vi "IO.vi"() -> ()   [LabVIEW 2020]
uses:
  Global_Variable/Global.vi
  Libraries/S7/S7.lvlib
panel:
  in  "输入轴旋转手动速度":sgl caption="手动速度" format="%#.3f"
  in  "输入轴旋转-正转":bool
  in  "输入轴旋转-反转":bool
  in  "输入轴旋转绝对位置":sgl caption="绝对位置" format="%#.3f"
  in  "输入轴旋转相对位置":sgl caption="相对位置" format="%#.3f"
  in  "输入轴旋转-绝对定位":bool
  in  "输入轴旋转-相对定位":bool
  out "输出轴旋转当前位置":sgl caption="当前位置" format="%#.3f"
  in  "输出轴旋转-反转":bool
  in  "输出轴旋转-正转":bool
  in  "输出轴旋转手动速度":sgl caption="手动速度" format="%#.3f"
  in  "工装移载手动速度":sgl caption="手动速度" format="%#.3f"
  in  "工装移载-正转":bool
  in  "工装移载-反转":bool
  in  "工装移载绝对位置":sgl caption="绝对位置" format="%#.3f"
  in  "工装移载相对位置":sgl caption="相对位置" format="%#.3f"
  in  "工装移载-绝对定位":bool
  in  "工装移载-相对定位":bool
  out "输入轴旋转状态":bool
  out "工装移载状态":bool
  out "输出轴旋转状态":bool
  in  "选项卡控件":enum32{"DI", "DO", "伺服"}(tab)
  out "I 1":T1
  out "I 3":T2
  out "I 2":T3
  out "I 0":T4
  out "I 4":T5
  out "I 5":T6
  in  "Q5":T7
  in  "Q4":T8
  in  "Q3":T9
  in  "Q2":T10
  in  "Q1":T11
  in  "Q0":T12
  out "电机角度":sgl caption="电机角度(°)" format="%#.3f"
  out "扭矩":sgl caption="扭矩(N)" format="%#.3f"
  out "拉压力":sgl caption="拉压力(N)" format="%#.3f"
  in  "输入轴移载相对位置":sgl caption="相对位置" format="%#.3f"
  in  "输入轴移载绝对位置":sgl caption="绝对位置" format="%#.3f"
  in  "拧紧轴手动速度":sgl caption="手动速度" format="%#.3f"
  out "输入轴移载状态":bool
  in  "输入轴移载-相对定位":bool
  in  "输入轴移载-绝对定位":bool
  in  "拧紧轴-反转":bool
  in  "拧紧轴-正转":bool
  out "输入轴旋转当前位置":sgl caption="当前位置" format="%#.3f"
  out "输入轴移载当前位置":sgl caption="当前位置" format="%#.3f"
  out "工装移载当前位置":sgl caption="当前位置" format="%#.3f"
  out "位移":sgl caption="电缸位移(MM)" format="%#.3f"
  in  "Q6":T13
  # "手动操作"
  # "输入轴旋转伺服"
  # "输出轴旋转伺服"
  # "工装移载伺服"
  # "输入轴移载伺服"
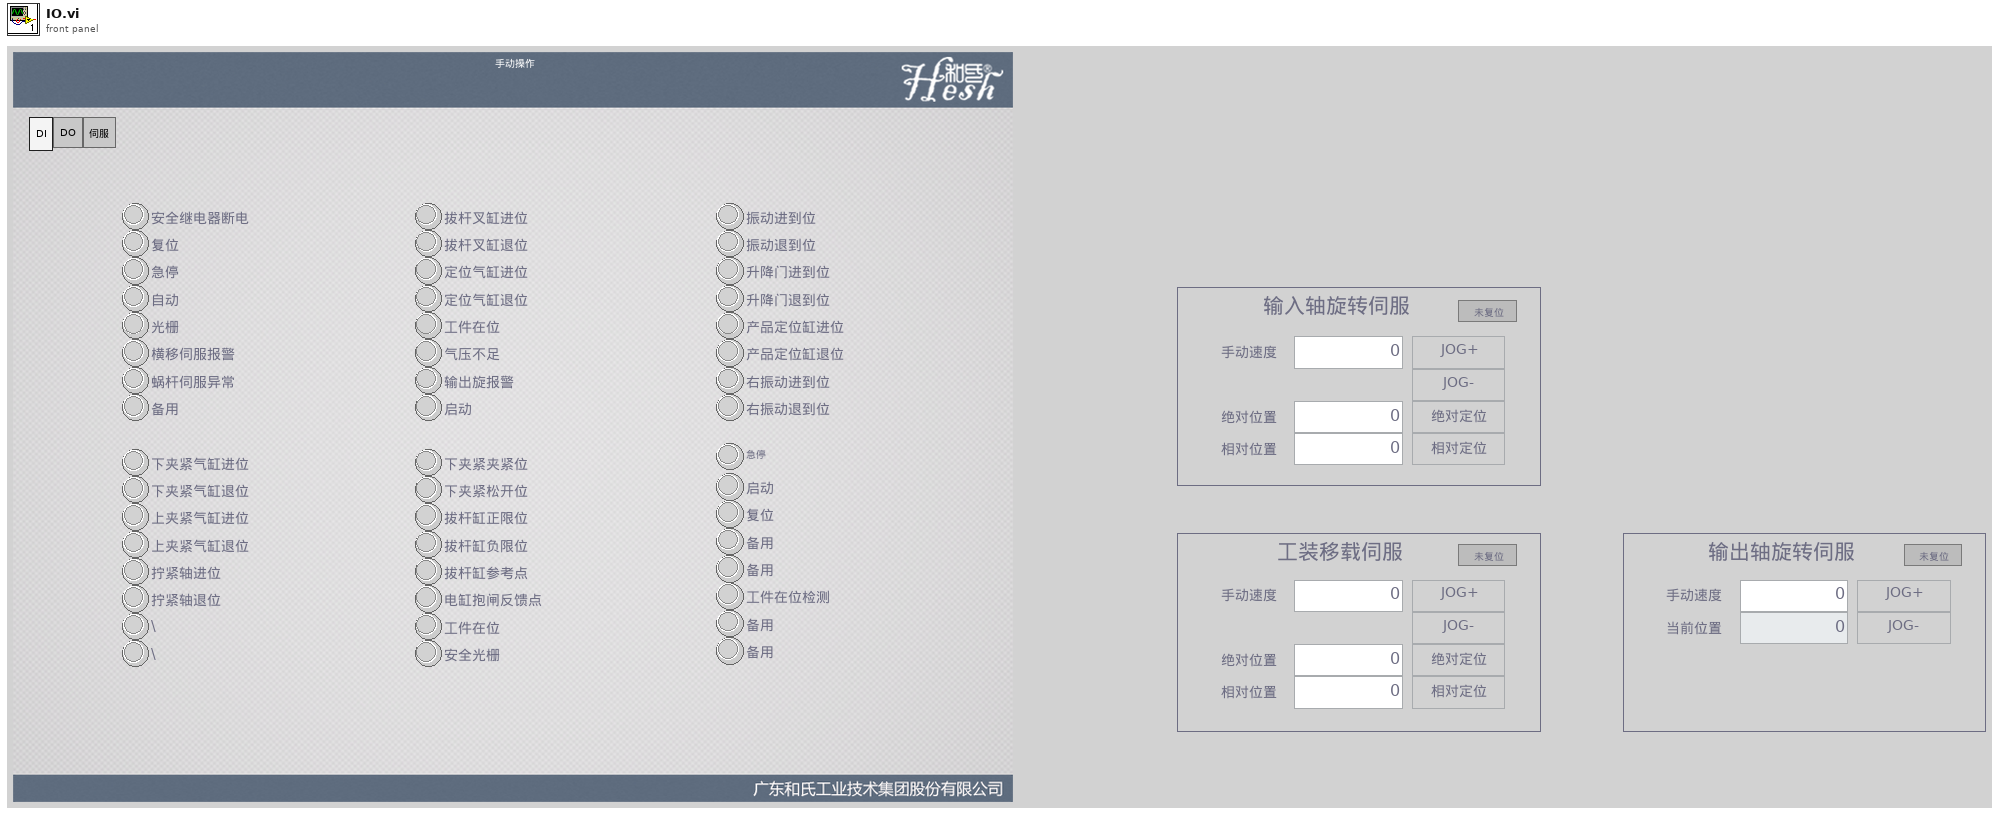
[diagram p1: front panel]
types:
  T1 = cluster{"下夹紧气缸进位":bool, "下夹紧气缸退位":bool, "上夹紧气缸进位":bool, "上夹紧气缸退位":bool, "拧紧轴进位":bool, "拧紧轴退位":bool, "\\":bool, "\\ ":bool}
  T2 = cluster{"下夹紧夹紧位":bool, "下夹紧松开位":bool, "拔杆缸正限位":bool, "拔杆缸负限位":bool, "拔杆缸参考点":bool, "电缸抱闸反馈点":bool, "工件在位":bool, "安全光栅":bool}
  T3 = cluster{"拔杆叉缸进位":bool, "拔杆叉缸退位":bool, "定位气缸进位":bool, "定位气缸退位":bool, "工件在位":bool, "气压不足":bool, "输出旋报警":bool, "启动":bool}
  T4 = cluster{"安全继电器断电":bool, "复位":bool, "急停":bool, "自动":bool, "光栅":bool, "横移伺服报警":bool, "蜗杆伺服异常":bool, "备用":bool}
  T5 = cluster{"振动进到位":bool, "振动退到位":bool, "升降门进到位":bool, "升降门退到位":bool, "产品定位缸进位":bool, "产品定位缸退位":bool, "右振动进到位":bool, "右振动退到位":bool}
  T6 = cluster{"急停":bool, "启动":bool, "复位":bool, "备用":bool, "备用":bool, "工件在位检测":bool, "备用":bool, "备用":bool}
  T7 = cluster{"产品定位缸进":bool, "产品定位缸退":bool, "右振动进":bool, "右振动退":bool, "高度适配轴复位":bool, "高度适配轴回原点":bool, "高度适配轴JOG+":bool, "高度适配轴JOG-":bool}
  T8 = cluster{"抱花键":bool, "摆臂进":bool, "摆臂退":bool, "升降门进":bool, "升降门退":bool, "振动":bool, "电机方向":bool, "电机控制":bool}
  T9 = cluster{"定位缸进":bool, "定位缸退":bool, "三色灯红":bool, "蜂鸣器":bool, "备用":bool, "switch":bool, "备用":bool, "备用":bool}
  T10 = cluster{"下气缸夹紧":bool, "下气缸松开":bool, "上气缸夹紧":bool, "上气缸松开":bool, "拧紧轴进":bool, "拧紧轴退":bool, "拔叉缸进":bool, "拔叉缸退":bool}
  T11 = cluster{"合格":bool, "不合格":bool, "/":bool, "/":bool, "/":bool, "/":bool, "/":bool, "/":bool}
  T12 = cluster{"轴1上":bool, "轴1下":bool, "轴2脉冲":bool, "轴2方向":bool, "蜂鸣器":bool, "黄灯":bool, "绿灯":bool, "红灯":bool}
  T13 = cluster{"输入轴移载上升":bool, "输入轴移载下降":bool, "输出轴移载上升":bool, "输出轴移载下降":bool, "输入轴左旋":bool, "输入轴右旋":bool, "输出轴左旋":bool, "输出轴右旋":bool}
  T14 = cluster{bool, bool, bool, bool, bool, bool, bool, bool}
  T15 = typedef "S7.lvlib/Read_Data (Reply Payload)--cluster.ctl" = cluster{"读取成功":bool, "数据":u32[], "Read_Data_error":errorcluster}
  T16 = cluster{"Boolean array[0]":bool, "Boolean array[1]":bool, "Boolean array[2]":bool, "Boolean array[3]":bool, "Boolean array[4]":bool, "Boolean array[5]":bool, "Boolean array[6]":bool, "Boolean array[7]":bool}
  T17 = cluster{"输入旋转位移":sgl, "输入移载位移":sgl, "工装移载位移":sgl, "输入编码位移":sgl, "扭矩":sgl, "输出扭矩(小)":sgl, "输出扭矩(大)":sgl, "吸收电流":sgl, "Factorysensor":sgl, "输出轴旋转角度":sgl, "输出轴移栽位移":sgl, "Factorysensor2":sgl}
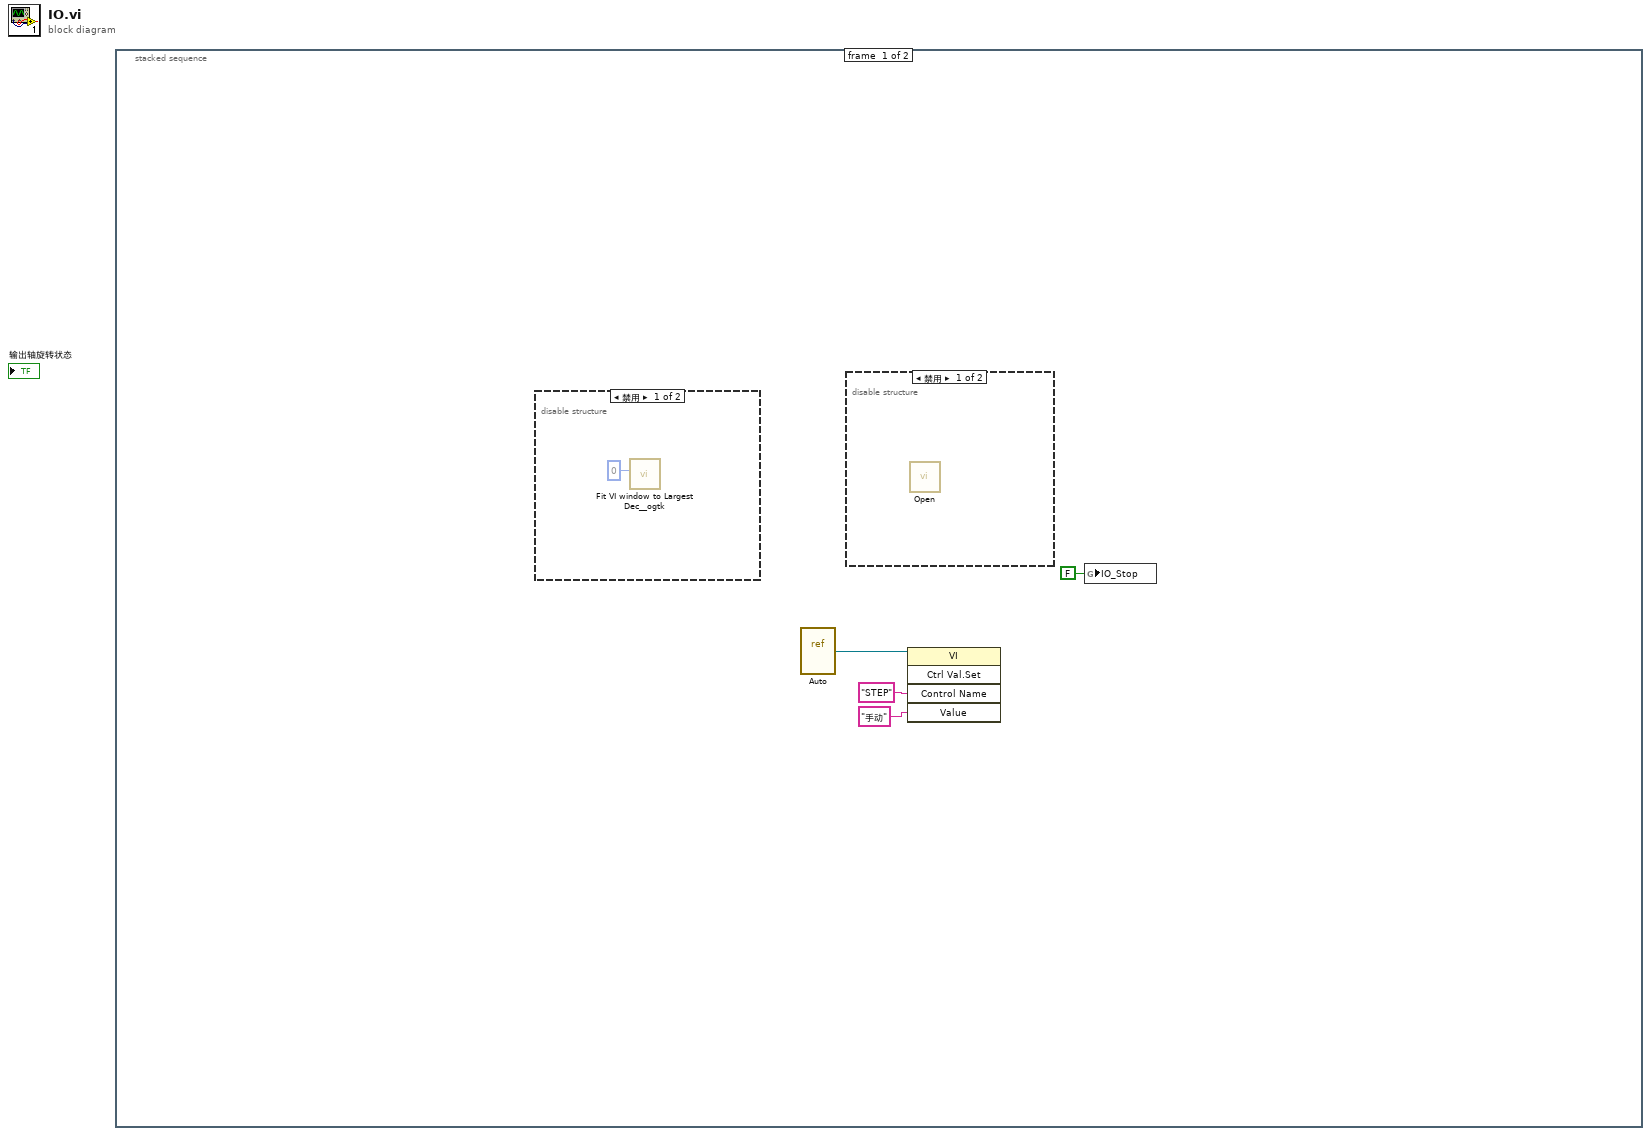
[diagram p0: block diagram]
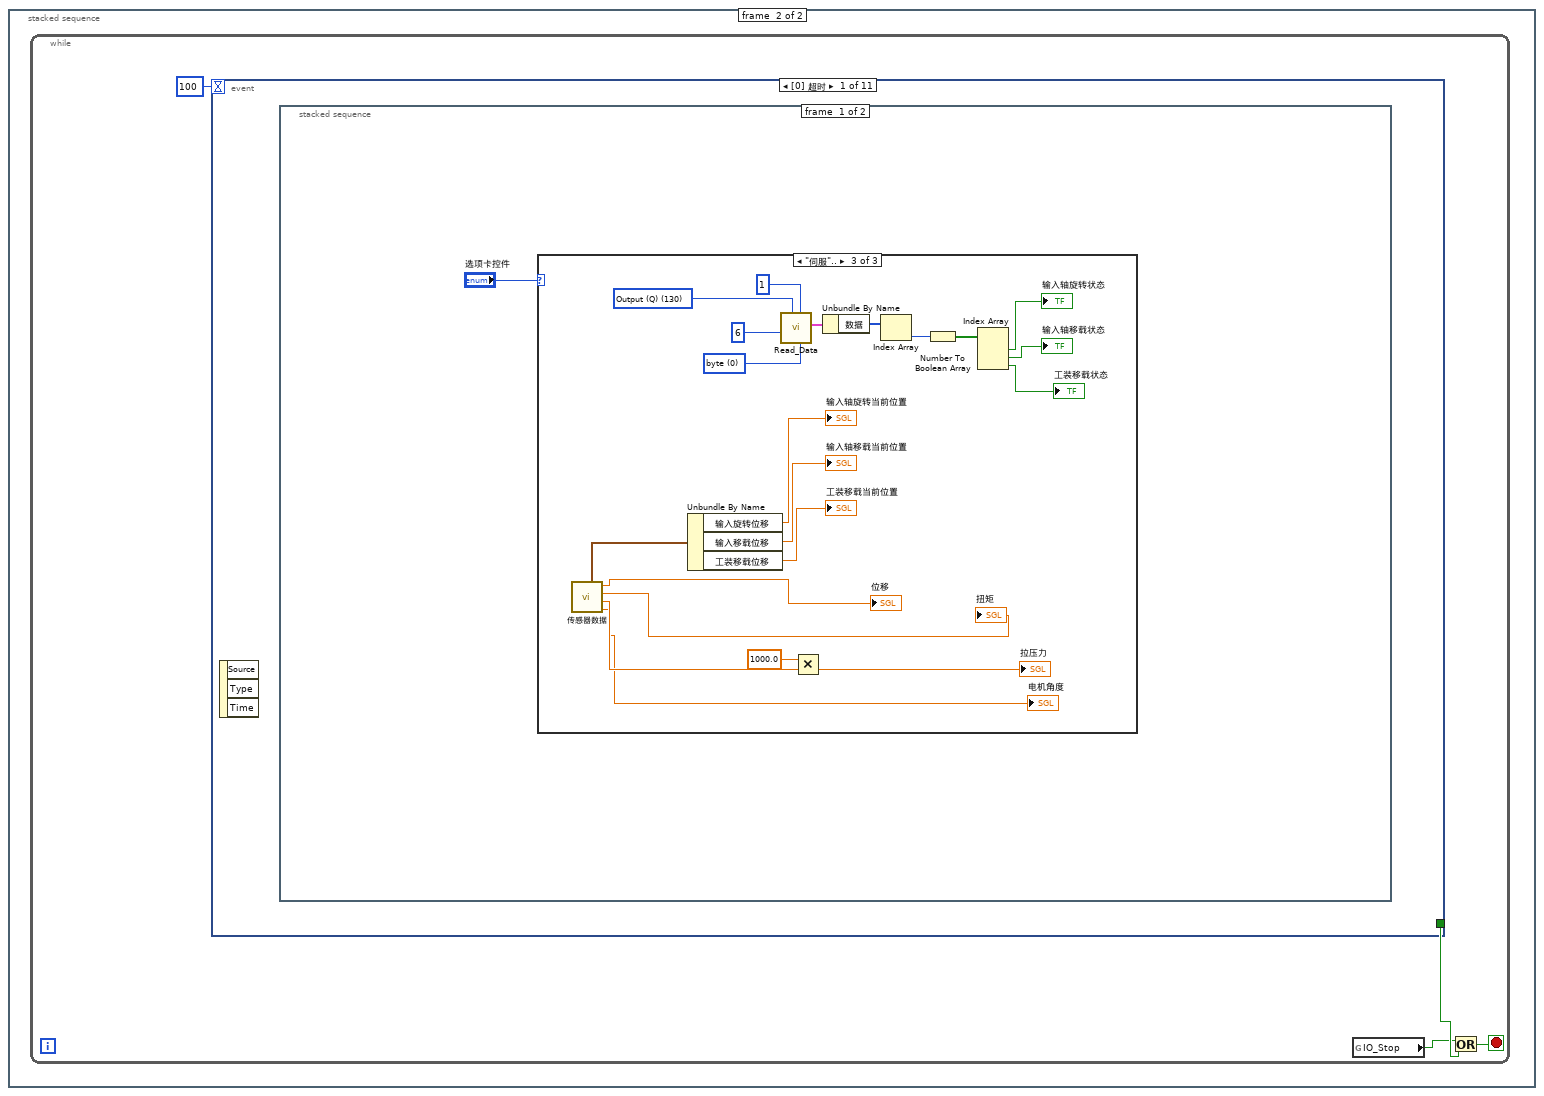
[diagram p4: hidden frame]
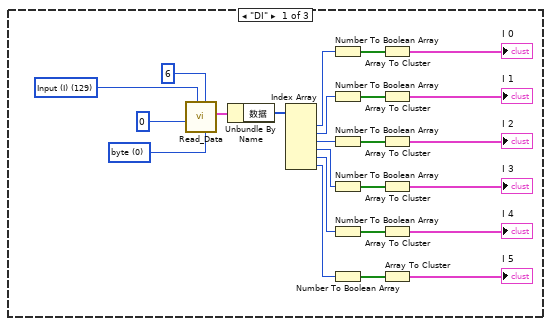
[diagram p5: hidden frame]
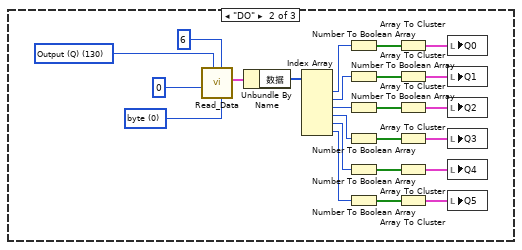
[diagram p6: hidden frame]
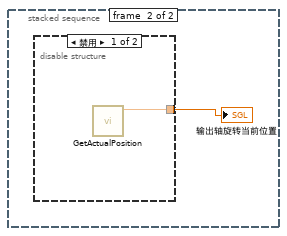
[diagram p7: hidden frame]
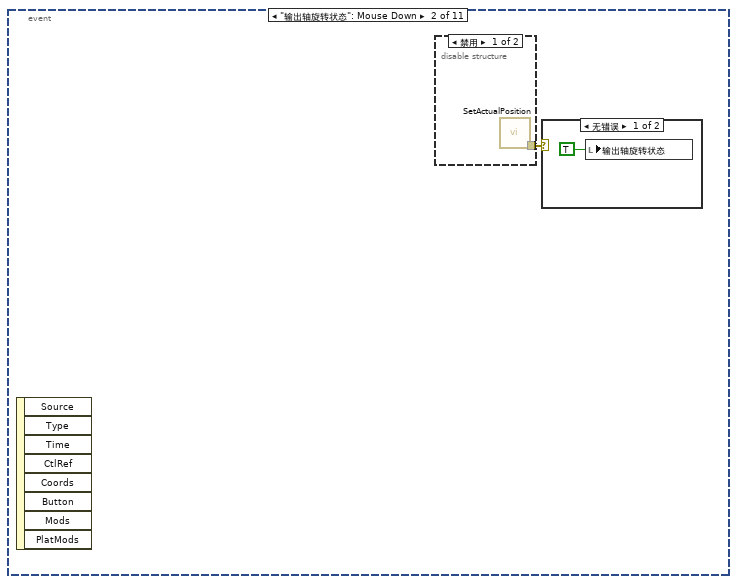
[diagram p9: hidden frame]
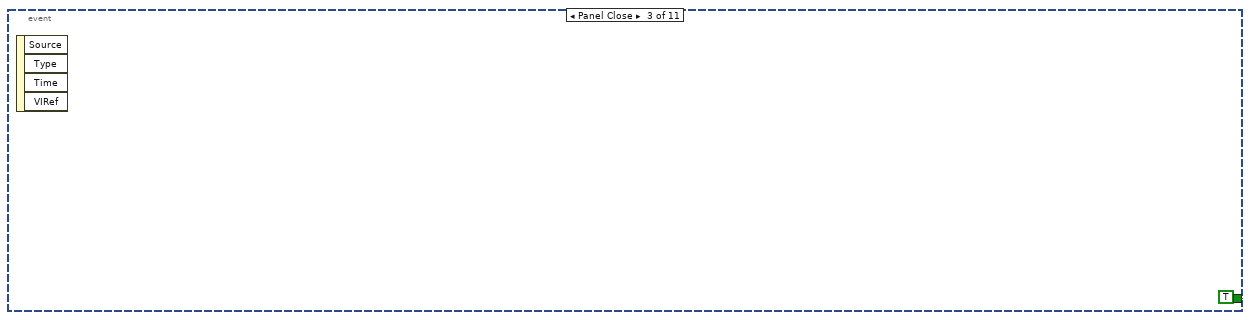
[diagram p12: hidden frame]
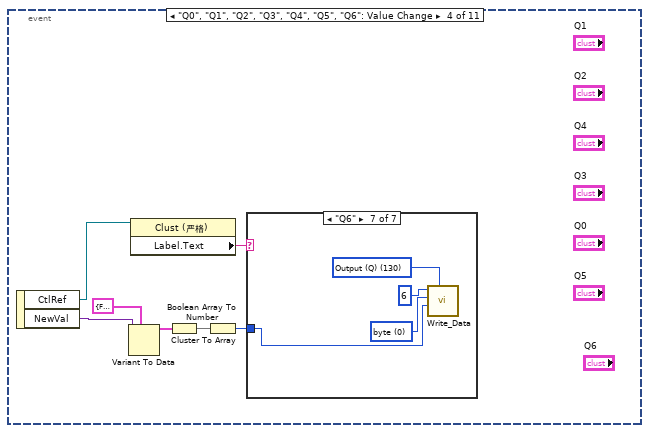
[diagram p13: hidden frame]
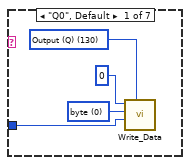
[diagram p14: hidden frame]
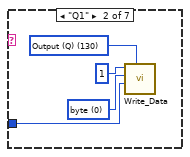
[diagram p15: hidden frame]
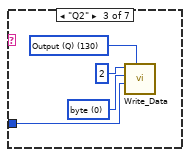
[diagram p16: hidden frame]
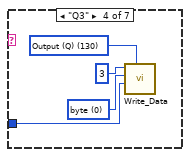
[diagram p17: hidden frame]
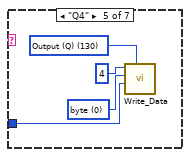
[diagram p18: hidden frame]
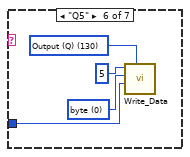
[diagram p19: hidden frame]
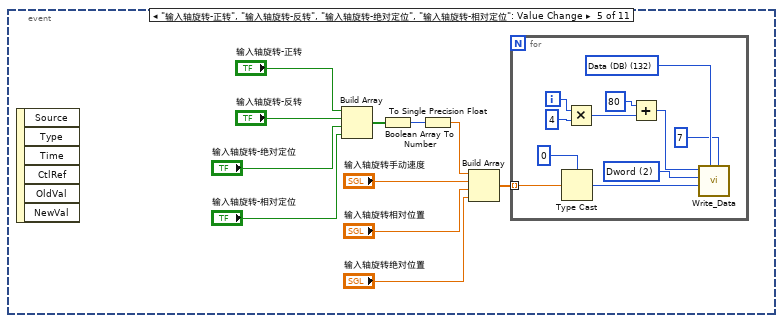
[diagram p20: hidden frame]
diagram:
  n1 = stacked-sequence {
    frame #0 {
      n2 = disable-structure shown="禁用" {
        frame Disabled {
          n3 = call <userlib>:"Fit VI window to Largest Dec__ogtk.vi"("border spacing (2 px)"=0) -> ()  [unwired: 5 in, 2 out]
        }
        frame Enabled {
        }
      }
      n4 = vi-ref "Auto.vi"() -> (w3:refnum<vi>)
      n5 = disable-structure shown="禁用" {
        frame Disabled {
          n6 = call "Open.vi"() -> ()  [unwired: 11 in, 1 out]
        }
        frame Enabled {
        }
      }
      n7 = invoke class="VI" method="Ctrl Val.Set"(reference=w3, "Control Name"="STEP" ("控件名"), "Value"="手动" ("控件名")) -> ()  [unwired: 2 in, 5 out]
      n8 = global write "Global.vi" "IO_Stop"(FALSE ("IO_Stop")) -> ()
    }
    frame #1 {
      n9 = while {
        stop <- w6 stop-if-true
        n10 = event shown="[0] 超时" {
          selector: _ -> [_ _ _ _ _ _ _ _ _ _ _]
          dyn-events: _ -> [_ _ _ _ _ _ _ _ _ _ _]
          timeout: 100 -> [_ _ _ _ _ _ _ _ _ _ _]
          tunnel: [_ _ TRUE _ _ _ _ _ _ _ _] -> w8
          event Timeout {
            n11 = event-data() -> ()  [unwired: 1 in, 3 out]
            n12 = stacked-sequence {
              frame #0 {
                n13 = case shown="\"伺服\".." "选项卡控件" {
                  frame "DI" {
                    w14 = u16 0 items=["byte", "word", "Dword"] ("数据类型")
                    w12 = u8 129 items=["I/O (P)"=128, "Input (I)"=129, "Output (Q)"=130, "Bit Memory (M)"=131, "Data (DB)"=132, "Instance Data (DI)"=133, "Local Data (L)"=134, "Predecessor Local Data (VL)"=135] ("寄存器类型")
                    n14 = call "Read_Data.vi"("数据类型"=w14, "读取长度"=u16 6, "寄存器类型"=w12, "起始地址"=u32 0) -> ("Reply Payload"=w16:T15)  [unwired: 5 in, 2 out]
                    n15 = Unbundle By Name(w16) -> ("数据"=w15:u32[])
                    n16 = Index Array(array=w15) -> (element #1=w28:u32, element #2=w30:u32, element #3=w29:u32, element #4=w25:u32, element #5=w24:u32, element #6=w23:u32)  [unwired: 6 in]
                    n17 = Number To Boolean Array(number=w28) -> (Boolean array=w27:bool[])
                    n18 = Number To Boolean Array(number=w30) -> (Boolean array=w26:bool[])
                    n19 = Number To Boolean Array(number=w29) -> (Boolean array=w22:bool[])
                    n20 = Number To Boolean Array(number=w25) -> (Boolean array=w20:bool[])
                    n21 = Number To Boolean Array(number=w24) -> (Boolean array=w18:bool[])
                    n22 = Number To Boolean Array(number=w23) -> (Boolean array=w17:bool[])
                    n23 = Array To Cluster(array=w27) -> (cluster=→"I 0":T16)
                    n24 = Array To Cluster(array=w26) -> (cluster=→"I 1":T16)
                    n25 = Array To Cluster(array=w22) -> (cluster=→"I 2":T16)
                    n26 = Array To Cluster(array=w20) -> (cluster=→"I 3":T16)
                    n27 = Array To Cluster(array=w18) -> (cluster=→"I 4":T16)
                    n28 = Array To Cluster(array=w17) -> (cluster=→"I 5":T16)
                  }
                  frame "DO" {
                    w38 = u16 0 items=["byte", "word", "Dword"] ("数据类型")
                    w36 = u8 130 items=["I/O (P)"=128, "Input (I)"=129, "Output (Q)"=130, "Bit Memory (M)"=131, "Data (DB)"=132, "Instance Data (DI)"=133, "Local Data (L)"=134, "Predecessor Local Data (VL)"=135] ("寄存器类型")
                    n29 = call "Read_Data.vi"("数据类型"=w38, "读取长度"=u16 6, "寄存器类型"=w36, "起始地址"=u32 0) -> ("Reply Payload"=w57:T15)  [unwired: 5 in, 2 out]
                    n30 = Unbundle By Name(w57) -> ("数据"=w58:u32[])
                    n31 = Index Array(array=w58) -> (element #1=w48:u32, element #2=w50:u32, element #3=w49:u32, element #4=w47:u32, element #5=w46:u32, element #6=w45:u32)  [unwired: 6 in]
                    n32 = Number To Boolean Array(number=w48) -> (Boolean array=w51:bool[])
                    n33 = Number To Boolean Array(number=w50) -> (Boolean array=w52:bool[])
                    n34 = Number To Boolean Array(number=w49) -> (Boolean array=w53:bool[])
                    n35 = Number To Boolean Array(number=w47) -> (Boolean array=w54:bool[])
                    n36 = Number To Boolean Array(number=w46) -> (Boolean array=w55:bool[])
                    n37 = Number To Boolean Array(number=w45) -> (Boolean array=w56:bool[])
                    n38 = Array To Cluster(array=w51) -> (cluster=w43:T16)
                    n39 = Array To Cluster(array=w52) -> (cluster=w44:T16)
                    n40 = Array To Cluster(array=w53) -> (cluster=w41:T16)
                    n41 = Array To Cluster(array=w54) -> (cluster=w42:T16)
                    n42 = Array To Cluster(array=w55) -> (cluster=w40:T16)
                    n43 = Array To Cluster(array=w56) -> (cluster=w39:T16)
                    n44 = local write "Q0"(w43) -> ()
                    n45 = local write "Q1"(w44) -> ()
                    n46 = local write "Q2"(w41) -> ()
                    n47 = local write "Q3"(w42) -> ()
                    n48 = local write "Q4"(w40) -> ()
                    n49 = local write "Q5"(w39) -> ()
                  }
                  frame "伺服".. {
                    w72 = u16 0 items=["byte", "word", "Dword"] ("数据类型")
                    w70 = u8 130 items=["I/O (P)"=128, "Input (I)"=129, "Output (Q)"=130, "Bit Memory (M)"=131, "Data (DB)"=132, "Instance Data (DI)"=133, "Local Data (L)"=134, "Predecessor Local Data (VL)"=135] ("寄存器类型")
                    n50 = call "传感器数据.vi"() -> ("电机角度"=→"电机角度":sgl, "拉压力"=w64:sgl, "扭矩"=→"扭矩":sgl, "电缸位移"=→"位移":sgl, "传感器读数"=w60:T17)  [unwired: 6 in, 1 out]
                    n51 = Unbundle By Name(w60) -> ("输入旋转位移"=→"输入轴旋转当前位置":sgl, "输入移载位移"=→"输入轴移载当前位置":sgl, "工装移载位移"=→"工装移载当前位置":sgl)
                    n52 = call "Read_Data.vi"("数据类型"=w72, "读取长度"=u16 1, "寄存器类型"=w70, "起始地址"=u32 6) -> ("Reply Payload"=w73:T15)  [unwired: 5 in, 2 out]
                    n53 = Multiply(x=sgl 1000.0, y=w64) -> (x*y=→"拉压力":sgl)
                    n54 = Unbundle By Name(w73) -> ("数据"=w74:u32[])
                    n55 = Index Array(array=w74) -> (element=w79:u32)  [unwired: 1 in]
                    n56 = Number To Boolean Array(number=w79) -> (Boolean array=w76:bool[])
                    n57 = Index Array(array=w76) -> (element #1=→"输入轴旋转状态":bool, element #2=→"输入轴移载状态":bool, element #3=→"工装移载状态":bool)  [unwired: 3 in]
                  }
                }
              }
              frame #1 {
                n58 = disable-structure shown="禁用" {
                  disable-tunnel: [w81 _] -> w80
                  frame Disabled {
                    n59 = call "GetActualPosition.vi"() -> ("Axis_ActualPosition(°)"=w81:dbl)  [unwired: 11 in]
                  }
                  frame Enabled {
                  }
                }
                "输出轴旋转当前位置" <- w80
              }
            }
          }
          event "输出轴旋转状态": Mouse Down {
            n60 = event-data() -> ()  [unwired: 1 in, 8 out]
            n61 = disable-structure shown="禁用" {
              disable-tunnel: [w83 _] -> w82
              frame Disabled {
                n62 = call "SetActualPosition.vi"() -> ("error out"=w83:errorcluster)  [unwired: 11 in]
              }
              frame Enabled {
              }
            }
            n63 = case shown="无错误" w82 {
              frame No Error {
                n64 = local write "输出轴旋转状态"(TRUE ("输出轴旋转状态")) -> ()
              }
              frame Error {
              }
            }
          }
          event Panel Close {
            n65 = event-data() -> ()  [unwired: 1 in, 4 out]
          }
          event "Q0", "Q1", "Q2", "Q3", "Q4", "Q5", "Q6": Value Change {
            n66 = event-data() -> ("CtlRef"=w87:refnum<vi>, "NewVal"=w91:variant)  [unwired: 1 in]
            n67 = Variant To Data(type=T14 {FALSE, FALSE, FALSE, FALSE, FALSE, FALSE, FALSE, FALSE}, Variant=w91) -> (data=w90:T14)  [unwired: 1 in, 1 out]
            n68 = property class="Clust (严格)"(reference=w87) -> ("Label.Text"=w86:string)  [unwired: 1 in, 2 out]
            n69 = Cluster To Array(cluster=w90) -> (array=w89:bool[])
            n70 = Boolean Array To Number(Boolean array=w89) -> (number=w88:u32)
            n71 = case shown="\"Q6\"" w86 {
              tunnel: w88 -> [w96 w100 w104 w108 w112 w116 w117]
              frame "Q0", Default {
                w94 = u16 0 items=["byte", "word", "Dword"] ("数据类型")
                w95 = u8 130 items=["I/O (P)"=128, "Input (I)"=129, "Output (Q)"=130, "Bit Memory (M)"=131, "Data (DB)"=132, "Instance Data (DI)"=133, "Local Data (L)"=134, "Predecessor Local Data (VL)"=135] ("寄存器类型")
                n72 = call "Write_Data.vi"("寄存器类型"=w95, "写入数据"=w96, "数据类型"=w94, "写入地址"=u32 0) -> ()  [unwired: 5 in, 3 out]
              }
              frame "Q1" {
                w98 = u16 0 items=["byte", "word", "Dword"] ("数据类型")
                w99 = u8 130 items=["I/O (P)"=128, "Input (I)"=129, "Output (Q)"=130, "Bit Memory (M)"=131, "Data (DB)"=132, "Instance Data (DI)"=133, "Local Data (L)"=134, "Predecessor Local Data (VL)"=135] ("寄存器类型")
                n73 = call "Write_Data.vi"("寄存器类型"=w99, "写入数据"=w100, "数据类型"=w98, "写入地址"=u32 1) -> ()  [unwired: 5 in, 3 out]
              }
              frame "Q2" {
                w102 = u16 0 items=["byte", "word", "Dword"] ("数据类型")
                w103 = u8 130 items=["I/O (P)"=128, "Input (I)"=129, "Output (Q)"=130, "Bit Memory (M)"=131, "Data (DB)"=132, "Instance Data (DI)"=133, "Local Data (L)"=134, "Predecessor Local Data (VL)"=135] ("寄存器类型")
                n74 = call "Write_Data.vi"("寄存器类型"=w103, "写入数据"=w104, "数据类型"=w102, "写入地址"=u32 2) -> ()  [unwired: 5 in, 3 out]
              }
              frame "Q3" {
                w106 = u16 0 items=["byte", "word", "Dword"] ("数据类型")
                w107 = u8 130 items=["I/O (P)"=128, "Input (I)"=129, "Output (Q)"=130, "Bit Memory (M)"=131, "Data (DB)"=132, "Instance Data (DI)"=133, "Local Data (L)"=134, "Predecessor Local Data (VL)"=135] ("寄存器类型")
                n75 = call "Write_Data.vi"("寄存器类型"=w107, "写入数据"=w108, "数据类型"=w106, "写入地址"=u32 3) -> ()  [unwired: 5 in, 3 out]
              }
              frame "Q4" {
                w110 = u16 0 items=["byte", "word", "Dword"] ("数据类型")
                w111 = u8 130 items=["I/O (P)"=128, "Input (I)"=129, "Output (Q)"=130, "Bit Memory (M)"=131, "Data (DB)"=132, "Instance Data (DI)"=133, "Local Data (L)"=134, "Predecessor Local Data (VL)"=135] ("寄存器类型")
                n76 = call "Write_Data.vi"("寄存器类型"=w111, "写入数据"=w112, "数据类型"=w110, "写入地址"=u32 4) -> ()  [unwired: 5 in, 3 out]
              }
              frame "Q5" {
                w114 = u16 0 items=["byte", "word", "Dword"] ("数据类型")
                w115 = u8 130 items=["I/O (P)"=128, "Input (I)"=129, "Output (Q)"=130, "Bit Memory (M)"=131, "Data (DB)"=132, "Instance Data (DI)"=133, "Local Data (L)"=134, "Predecessor Local Data (VL)"=135] ("寄存器类型")
                n77 = call "Write_Data.vi"("寄存器类型"=w115, "写入数据"=w116, "数据类型"=w114, "写入地址"=u32 5) -> ()  [unwired: 5 in, 3 out]
              }
              frame "Q6" {
                w119 = u16 0 items=["byte", "word", "Dword"] ("数据类型")
                w120 = u8 130 items=["I/O (P)"=128, "Input (I)"=129, "Output (Q)"=130, "Bit Memory (M)"=131, "Data (DB)"=132, "Instance Data (DI)"=133, "Local Data (L)"=134, "Predecessor Local Data (VL)"=135] ("寄存器类型")
                n78 = call "Write_Data.vi"("寄存器类型"=w120, "写入数据"=w117, "数据类型"=w119, "写入地址"=u32 6) -> ()  [unwired: 5 in, 3 out]
              }
            }
          }
          event "输入轴旋转-正转", "输入轴旋转-反转", "输入轴旋转-绝对定位", "输入轴旋转-相对定位": Value Change {
            n79 = event-data() -> ()  [unwired: 1 in, 6 out]
            n80 = Build Array("输入轴旋转-正转", "输入轴旋转-反转", "输入轴旋转-绝对定位", "输入轴旋转-相对定位") -> (w130:bool[])
            n81 = Boolean Array To Number(Boolean array=w130) -> (number=w129:u32)
            n82 = To Single Precision Float(number=w129) -> (single precision float=w131:sgl)
            n83 = Build Array(w131, "输入轴旋转手动速度", "输入轴旋转相对位置", "输入轴旋转绝对位置") -> (w128:sgl[])
            n84 = for {
              tunnel: w128 -> [w137] mode=indexing
              i -> [w134]
              w139 = u16 2 items=["byte", "word", "Dword"] ("数据类型")
              w142 = u8 132 items=["I/O (P)"=128, "Input (I)"=129, "Output (Q)"=130, "Bit Memory (M)"=131, "Data (DB)"=132, "Instance Data (DI)"=133, "Local Data (L)"=134, "Predecessor Local Data (VL)"=135] ("寄存器类型")
              n85 = Type Cast(type=u32 0, x=w137) -> (*(type *) &x=w136:u32)
              n86 = Multiply(x=w134, y=u32 4) -> (x*y=w133:u32)
              n87 = Add(x=u32 80 ("写入地址"), y=w133) -> (x+y=w132:u32)
              n88 = call "Write_Data.vi"("DB #"=u16 7, "寄存器类型"=w142, "写入数据"=w136, "数据类型"=w139, "写入地址"=w132) -> ()  [unwired: 4 in, 3 out]
            }
          }
          event "拧紧轴-正转", "拧紧轴-反转", "输入轴移载-绝对定位", "输入轴移载-相对定位": Value Change {
            n89 = event-data() -> ()  [unwired: 1 in, 6 out]
            n90 = Build Array("拧紧轴-正转", "拧紧轴-反转", "输入轴移载-绝对定位", "输入轴移载-相对定位") -> (w152:bool[])
            n91 = Boolean Array To Number ("布尔数组至数值转换")(Boolean array=w152) -> (number=w151:u32)
            n92 = To Single Precision Float ("转换为单精度浮点数")(number=w151) -> (single precision float=w153:sgl)
            n93 = Build Array(w153, "拧紧轴手动速度", "输入轴移载相对位置", "输入轴移载绝对位置") -> (w150:sgl[])
            n94 = for {
              tunnel: w150 -> [w162] mode=indexing
              i -> [w160]
              w155 = u16 2 items=["byte", "word", "Dword"] ("数据类型")
              w157 = u8 132 items=["I/O (P)"=128, "Input (I)"=129, "Output (Q)"=130, "Bit Memory (M)"=131, "Data (DB)"=132, "Instance Data (DI)"=133, "Local Data (L)"=134, "Predecessor Local Data (VL)"=135] ("寄存器类型")
              n95 = Type Cast(type=u32 0, x=w162) -> (*(type *) &x=w154:u32)
              n96 = Multiply(x=w160, y=u32 4) -> (x*y=w159:u32)
              n97 = Add(x=u32 64 ("写入地址"), y=w159) -> (x+y=w156:u32)
              n98 = call "Write_Data.vi"("DB #"=u16 7, "寄存器类型"=w157, "写入数据"=w154, "数据类型"=w155, "写入地址"=w156) -> ()  [unwired: 4 in, 3 out]
            }
          }
          event "输出轴旋转-正转", "输出轴旋转-反转": Value Change {
            n99 = event-data() -> ()  [unwired: 1 in, 1 out]
            n100 = Build Array("输出轴旋转-正转", "输出轴旋转-反转") -> (w166:bool[])
            n101 = Boolean Array To Number(Boolean array=w166) -> (number=w165:u32)
            n102 = case shown="2" w165 {
              tunnel: "输出轴旋转手动速度" -> [_ w176 w177]
              tunnel: [sgl 0.0 ("输出轴旋转手动速度") w175 w177] -> w169
              frame 0, Default {
              }
              frame 2 {
                n103 = Negate(x=w176) -> (-x=w175:sgl)
              }
              frame 1 {
              }
            }
            n104 = disable-structure shown="禁用" {
              disable-tunnel: 100.0 ("Max Torque") -> [w173 _]
              disable-tunnel: w169 -> [w172 _]
              frame Disabled {
                n105 = call-poly "模式选择.vi"("Max Torque"=w173, "Velocity"=w172) -> ()  [unwired: 9 in, 1 out]
              }
              frame Enabled {
              }
            }
          }
          event "输入轴旋转状态": Mouse Down {
            w180 = u16 2 items=["byte", "word", "Dword"] ("数据类型")
            w182 = u8 132 items=["I/O (P)"=128, "Input (I)"=129, "Output (Q)"=130, "Bit Memory (M)"=131, "Data (DB)"=132, "Instance Data (DI)"=133, "Local Data (L)"=134, "Predecessor Local Data (VL)"=135] ("寄存器类型")
            n106 = event-data() -> ()  [unwired: 1 in, 1 out]
            n107 = Type Cast(type=u32 0, x=sgl 16.0) -> (*(type *) &x=w184:u32)
            n108 = call "Write_Data.vi"("DB #"=u16 7, "寄存器类型"=w182, "写入数据"=w184, "数据类型"=w180, "写入地址"=u32 80) -> ()  [unwired: 4 in, 3 out]
          }
          event "输入轴移载状态": Mouse Down {
            w185 = u16 2 items=["byte", "word", "Dword"] ("数据类型")
            w188 = u8 132 items=["I/O (P)"=128, "Input (I)"=129, "Output (Q)"=130, "Bit Memory (M)"=131, "Data (DB)"=132, "Instance Data (DI)"=133, "Local Data (L)"=134, "Predecessor Local Data (VL)"=135] ("寄存器类型")
            n109 = event-data() -> ()  [unwired: 1 in, 1 out]
            n110 = Type Cast(type=u32 0, x=sgl 16.0) -> (*(type *) &x=w191:u32)
            n111 = call "Write_Data.vi"("DB #"=u16 7, "寄存器类型"=w188, "写入数据"=w191, "数据类型"=w185, "写入地址"=u32 64) -> ()  [unwired: 4 in, 3 out]
          }
          event "工装移载状态": Mouse Down {
            w192 = u16 2 items=["byte", "word", "Dword"] ("数据类型")
            w195 = u8 132 items=["I/O (P)"=128, "Input (I)"=129, "Output (Q)"=130, "Bit Memory (M)"=131, "Data (DB)"=132, "Instance Data (DI)"=133, "Local Data (L)"=134, "Predecessor Local Data (VL)"=135] ("寄存器类型")
            n112 = event-data() -> ()  [unwired: 1 in, 1 out]
            n113 = Type Cast(type=u32 0, x=sgl 16.0) -> (*(type *) &x=w198:u32)
            n114 = call "Write_Data.vi"("DB #"=u16 7, "寄存器类型"=w195, "写入数据"=w198, "数据类型"=w192, "写入地址"=u32 104) -> ()  [unwired: 4 in, 3 out]
          }
          event "工装移载-正转", "工装移载-反转", "工装移载-绝对定位", "工装移载-相对定位": Value Change {
            n115 = event-data() -> ()  [unwired: 1 in, 6 out]
            n116 = Build Array("工装移载-正转", "工装移载-反转", "工装移载-绝对定位", "工装移载-相对定位") -> (w205:bool[])
            n117 = Boolean Array To Number(Boolean array=w205) -> (number=w204:u32)
            n118 = To Single Precision Float(number=w204) -> (single precision float=w203:sgl)
            n119 = Build Array(w203, "工装移载手动速度", "工装移载相对位置", "工装移载绝对位置") -> (w201:sgl[])
            n120 = for {
              tunnel: w201 -> [w215] mode=indexing
              i -> [w212]
              w217 = u16 2 items=["byte", "word", "Dword"] ("数据类型")
              w220 = u8 132 items=["I/O (P)"=128, "Input (I)"=129, "Output (Q)"=130, "Bit Memory (M)"=131, "Data (DB)"=132, "Instance Data (DI)"=133, "Local Data (L)"=134, "Predecessor Local Data (VL)"=135] ("寄存器类型")
              n121 = Type Cast(type=u32 0, x=w215) -> (*(type *) &x=w214:u32)
              n122 = Multiply(x=w212, y=u32 4) -> (x*y=w211:u32)
              n123 = Add(x=u32 104 ("写入地址"), y=w211) -> (x+y=w210:u32)
              n124 = call "Write_Data.vi"("DB #"=u16 7, "寄存器类型"=w220, "写入数据"=w214, "数据类型"=w217, "写入地址"=w210) -> ()  [unwired: 4 in, 3 out]
            }
          }
        }
        n125 = global read "Global.vi" "IO_Stop"() -> (w7:bool)
        n126 = Or(x=w7, y=w8) -> (x .or. y?=w6:bool)
      }
    }
  }
